vi "String Array 2 String.vi"(0 "Substrings":string[](array[string]), 1 "Delimiter (\",\")":string=",") -> (2 "String":string)   [LabVIEW 2015, in "CS++Utilities.lvlib"]
doc: "This VI converts an array of strings to a string with substrings separated by <b>Delimiter</b>."
uses:
  CS++Utilities.lvlib
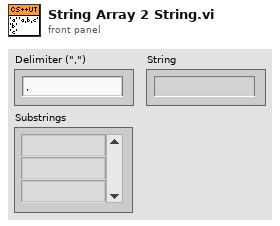
[diagram p1: front panel]
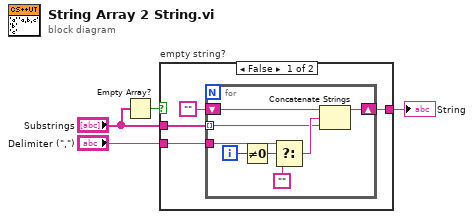
[diagram p0: block diagram]
diagram:
  n1 = Empty Array?(array="Substrings") -> (empty?=w3:bool)
  n2 = case "empty string?" shown="False" w3 {
    tunnel: "Delimiter (\",\")" -> [w7 _]
    tunnel: "Substrings" -> [w8 _]
    tunnel: [w5 _] -> w1
    frame False {
      n3 = for {
        tunnel: w8 -> [w11] mode=indexing
        tunnel: w7 -> [w15]
        shift-right: [w10] -> w5
        shift-left: "" -> [w9]
        i -> [w16]
        n4 = Not Equal To 0?(x=w16) -> (x != 0?=w14:bool)
        n5 = Select(t=w15, s=w14, f="") -> (s? t:f=w12:string)
        n6 = Concatenate Strings(w9, w12, w11) -> (w10:string)
      }
    }
    frame True {
    }
  }
  "String" <- w1
